vi "Scan.vi"(3 "SN":string) -> ()   [LabVIEW 2013]
uses:
  Global constant.vi
panel:
  in  "OK Button":bool
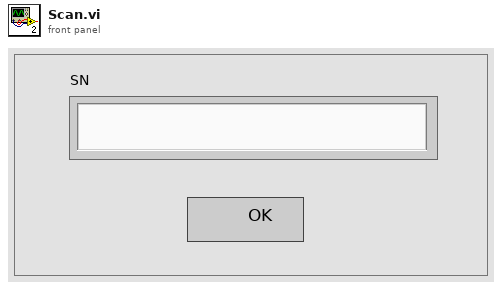
[diagram p1: front panel]
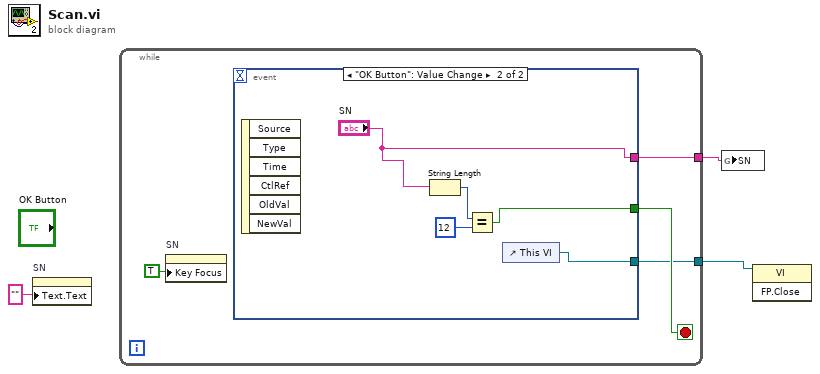
[diagram p0: block diagram]
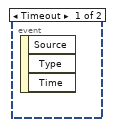
[diagram p2: hidden frame]
diagram:
  n1 = property on="SN" class="Str"("Text.Text"="") -> ()  [unwired: 2 in, 2 out]
  n2 = while {
    tunnel: [w5] -> w2
    tunnel: [w4] -> w1
    stop <- w7 stop-if-true
    n3 = property on="SN" class="Str"("Key Focus"=TRUE) -> ()  [unwired: 2 in, 2 out]
    n4 = event shown="[1] \"OK Button\": Value Change" {
      selector: _ -> [_ _]
      dyn-events: _ -> [_ _]
      timeout: _ -> [_ _]
      tunnel: [_ w10] -> w7
      tunnel: [_ "SN"] -> w5
      tunnel: [_ w9] -> w4
      event Timeout {
        n5 = event-data() -> ()  [unwired: 1 in, 3 out]
      }
      event "OK Button": Value Change {
        n6 = event-data() -> ()  [unwired: 1 in, 6 out]
        n7 = String Length(string="SN") -> (length=w12:i32)
        n8 = Equal?(x=w12, y=12) -> (x = y?=w10:bool)
        n9 = control-ref of="This VI"() -> (w9:refnum<vi>)
      }
    }
  }
  n10 = global write "Global constant.vi" "SN"(w2) -> ()
  n11 = invoke class="VI" method="FP.Close"(reference=w1) -> ()  [unwired: 2 in, 3 out]
